vi "SetTemp.vi"(3 "error in (no error)":errorcluster, 4 "Set Temperature":dbl format="%#_13g", 5 "VISA resource name":refnum<visa-resource-name>) -> (0 "error out":errorcluster)   [LabVIEW 2017]
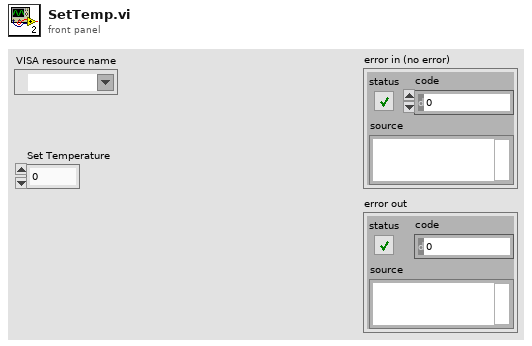
[diagram p1: front panel]
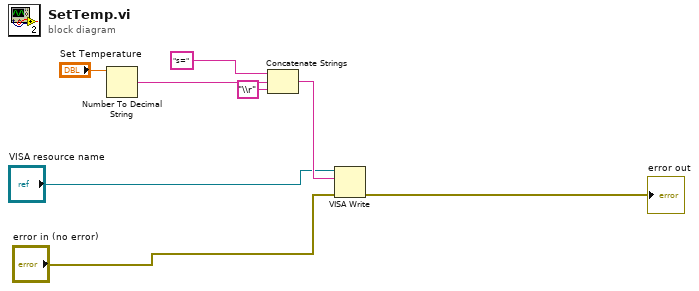
[diagram p0: block diagram]
diagram:
  n1 = Number To Decimal String(number="Set Temperature") -> (decimal integer string=w6:string)  [unwired: 1 in]
  n2 = Concatenate Strings("s=" ("write buffer"), w6, "\\r" ("string")) -> (w8:string)
  n3 = VISA Write(VISA resource name="VISA resource name", write buffer=w8, error in (no error)="error in (no error)") -> (error out=→"error out":errorcluster)  [unwired: 2 out]
